vi "Endpoint.vi"(6 "abort (F)":bool, 9 "element in":T2={"Temp. Sensirion"=0.01, "Hum. Sensirion"=0.01, "Temp. Switch Matrix"=0.01, "Hum. Switch Matrix"=0.01, "Temp. Probecard"=0.01, "Hum. Probecard"=0.01} {"Hum. Probecard" format="%#_13g"; "Temp. Probecard" format="%#_13g"; "Hum. Switch Matrix" format="%#_13g"; "Temp. Switch Matrix" format="%#_13g"; "Hum. Sensirion" format="%#_13g"; "Temp. Sensirion" format="%#_13g"}) -> (0 "missed":i32, 1 "element out":T2={"Temp. Sensirion"=0.01, "Hum. Sensirion"=0.01, "Temp. Switch Matrix"=0.01, "Hum. Switch Matrix"=0.01, "Temp. Probecard"=0.01, "Hum. Probecard"=0.01} {"Hum. Probecard" format="%#_13g"; "Temp. Probecard" format="%#_13g"; "Hum. Switch Matrix" format="%#_13g"; "Temp. Switch Matrix" format="%#_13g"; "Hum. Sensirion" format="%#_13g"; "Temp. Sensirion" format="%#_13g"}, 3 "channel out":T1, 4 "aborted?":bool)   [LabVIEW 2020, in "Tag-t'data_env.ctl'.lvlib"]
uses:
  <extravilib>/ChannelInstances/Tag-t'data_env.ctl'.lvlib
  Desktop/HexDAQ/src/data_env.ctl
  <extravilib>/ChannelInstances/Tag-t'data_env.ctl'/))Channel.ctl
  <extravilib>/ChannelInstances/Tag-t'data_env.ctl'/ChannelOp.ctl
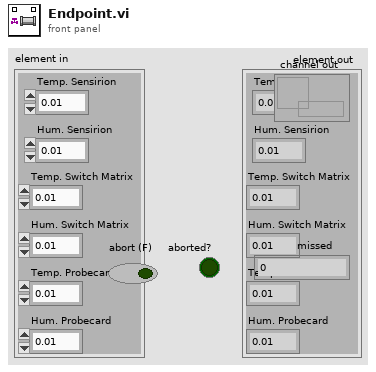
[diagram p1: front panel]
types:
  T1 = typedef "Tag-t'data_env.ctl'.lvlib/))Channel.ctl" = refnum<queue>
  T2 = typedef "data_env.ctl" = cluster{"Temp. Sensirion":dbl, "Hum. Sensirion":dbl, "Temp. Switch Matrix":dbl, "Hum. Switch Matrix":dbl, "Temp. Probecard":dbl, "Hum. Probecard":dbl}
  T3 = typedef "Tag-t'data_env.ctl'.lvlib/ChannelOp.ctl" = enum16{"init", "write", "read", "probe"}
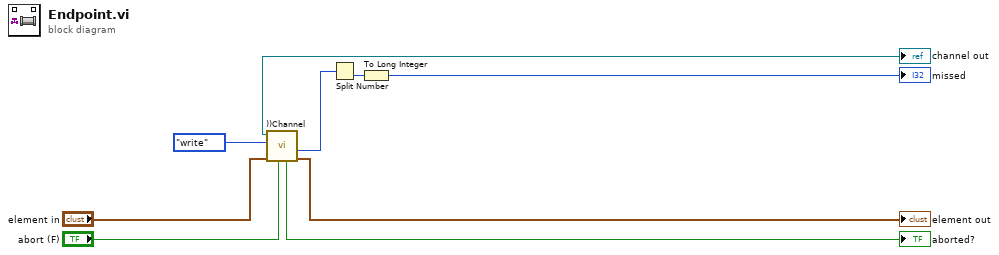
[diagram p0: block diagram]
diagram:
  n1 = call <extravilib>:"))Channel.vi"("abort (F)"="abort (F)", "element in"="element in", "channelOp"=ChannelOp."write", "channel in"="channel out") -> ("element out"=→"element out":T2, "sequence"=w3:u64, "aborted?"=→"aborted?":bool)  [unwired: 2 in, 3 out]
  n2 = Split Number(x=w3) -> (lo(x)=w1:u32)  [unwired: 1 out]
  n3 = To Long Integer(number=w1) -> (32bit integer=→"missed":i32)
